vi "rpr -- list of _a files.vi"(6 "suffix":string="a", 11 "9w folder path":path=path "C:/data/RUS/Experiment/ProbeTest/Probe10/YBCO_5/sweep2/9w") -> (0 "Array":string[](array[string]))   [LabVIEW 2014]
uses:
  <vilib>/regexp/Match Regular Expression.xnode
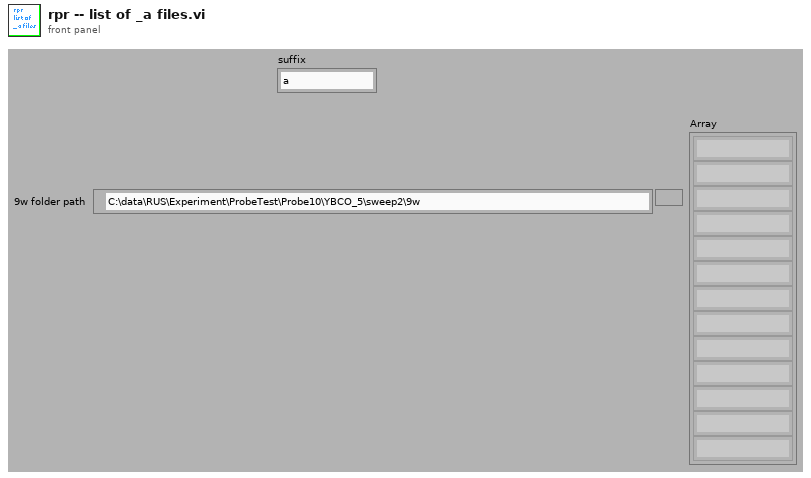
[diagram p1: front panel]
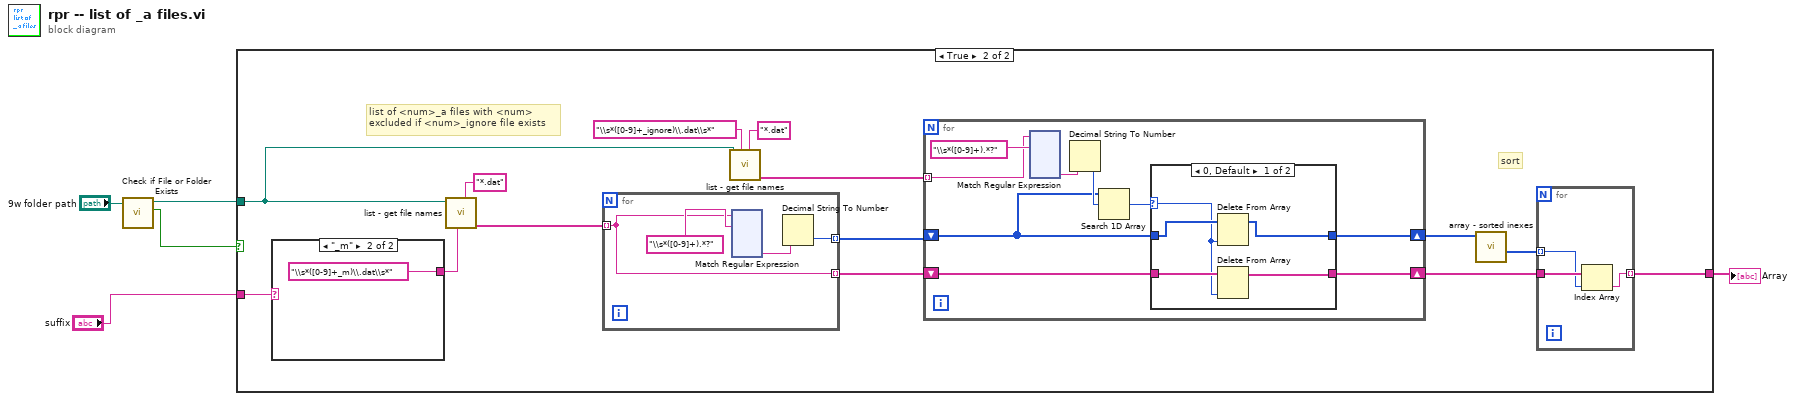
[diagram p0: block diagram]
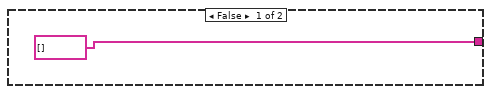
[diagram p2: hidden frame]
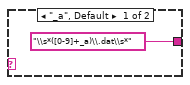
[diagram p3: hidden frame]
diagram:
  n1 = call <vilib>:"Check if File or Folder Exists.vi"("path"="9w folder path") -> ("file or folder exists?"=w3:bool, "dup path"=w4:path)  [unwired: 8 in, 1 out]
  n2 = case shown="True" w3 {
    tunnel: w4 -> [_ w12]
    tunnel: [string[] [] w8] -> w2
    tunnel: "suffix" -> [_ w7]
    frame False {
    }
    frame True {
      # "sort"
      # "list of <num>_a files with <num> \nexcluded if <num>_ignore file exists"
      n3 = case shown="\"_m\"" w7 {
        tunnel: ["\\s*([0-9]+_a)\\.dat\\s*" ("regular expression") "\\s*([0-9]+_m)\\.dat\\s*" ("regular expression")] -> w19
        frame "_a", Default {
        }
        frame "_m" {
        }
      }
      n4 = call "list - get file names.vi"("extension filter"="*.dat" ("pattern"), "regular expression"=w19, "folder path"=w12) -> ("Array"=w16:string[])  [unwired: 7 in, 1 out]
      n5 = for {
        tunnel: w16 -> [w155] mode=indexing
        tunnel: [w156] -> w14 mode=indexing
        tunnel: [w155] -> w13 mode=indexing
        n6 = xnode "Match Regular Expression"("input string"=w155, "regular expression"="\\s*([0-9]+).*?") -> ("submatch 1"=w157:string)  [unwired: 4 in, 5 out]
        n7 = Decimal String To Number(string=w157) -> (number=w156:i32)  [unwired: 2 in, 1 out]
      }
      n8 = call "list - get file names.vi"("extension filter"="*.dat" ("pattern"), "regular expression"="\\s*([0-9]+_ignore)\\.dat\\s*", "folder path"=w12) -> ("Array"=w15:string[])  [unwired: 7 in, 1 out]
      n9 = for {
        tunnel: w15 -> [w32] mode=indexing
        shift-right: [w29] -> w11
        shift-left: w14 -> [w28]
        shift-right: [w27] -> w9
        shift-left: w13 -> [w26]
        n10 = xnode "Match Regular Expression"("input string"=w32, "regular expression"="\\s*([0-9]+).*?") -> ("submatch 1"=w34:string)  [unwired: 4 in, 5 out]
        n11 = Decimal String To Number(string=w34) -> (number=w31:i32)  [unwired: 2 in, 1 out]
        n12 = Search 1D Array(1D array=w28, element=w31) -> (index of element=w30:i32)  [unwired: 1 in]
        n13 = case shown="0, Default" w30 {
          selector: w30 -> [w36 _]
          tunnel: [w38 w41] -> w29
          tunnel: w28 -> [w39 w41]
          tunnel: [w35 w40] -> w27
          tunnel: w26 -> [w37 w40]
          frame 0, Default {
            n14 = Delete From Array(array=w39, index=w36) -> (array with subset deleted=w38:i32[])  [unwired: 1 in, 1 out]
            n15 = Delete From Array(array=w37, index=w36) -> (array with subset deleted=w35:string[])  [unwired: 1 in, 1 out]
          }
          frame -1 {
          }
        }
      }
      n16 = call "array - sorted inexes.vi"("x"=w11) -> ("index array"=w10:i32[])  [unwired: 9 in, 1 out]
      n17 = for {
        tunnel: w10 -> [w24] mode=indexing
        tunnel: w9 -> [w25]
        tunnel: [w23] -> w8 mode=indexing
        n18 = Index Array(array=w25, index=w24) -> (element=w23:string)
      }
    }
  }
  "Array" <- w2
